vi "Digital Input Read.vi"(8 "error in (no error)":errorcluster, 11 "NI Digital Input in":refnum<class "NI Digital Input.lvclass">) -> (0 "error out":errorcluster, 2 "data":bool[](array[boolean]), 3 "NI Digital Input out":refnum<class "NI Digital Input.lvclass">)   [LabVIEW 2023, in "HardwareAbstractionLayer_LVOOP.lvlib" / "NI Digital Input.lvclass"]
uses:
  NI Digital Input.lvclass
  NI Digital Input.lvclass/NI Digital Input.ctl
  <vilib>/DAQmx/read.llb/DAQmx Read (Digital 1D Bool NChan 1Samp 1Line).vi
  <vilib>/DAQmx/miscellaneous.llb/DAQmx Fill In Error Info.vi
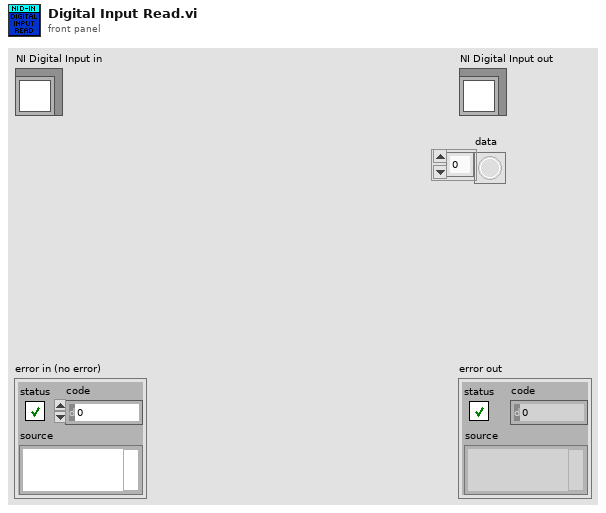
[diagram p1: front panel]
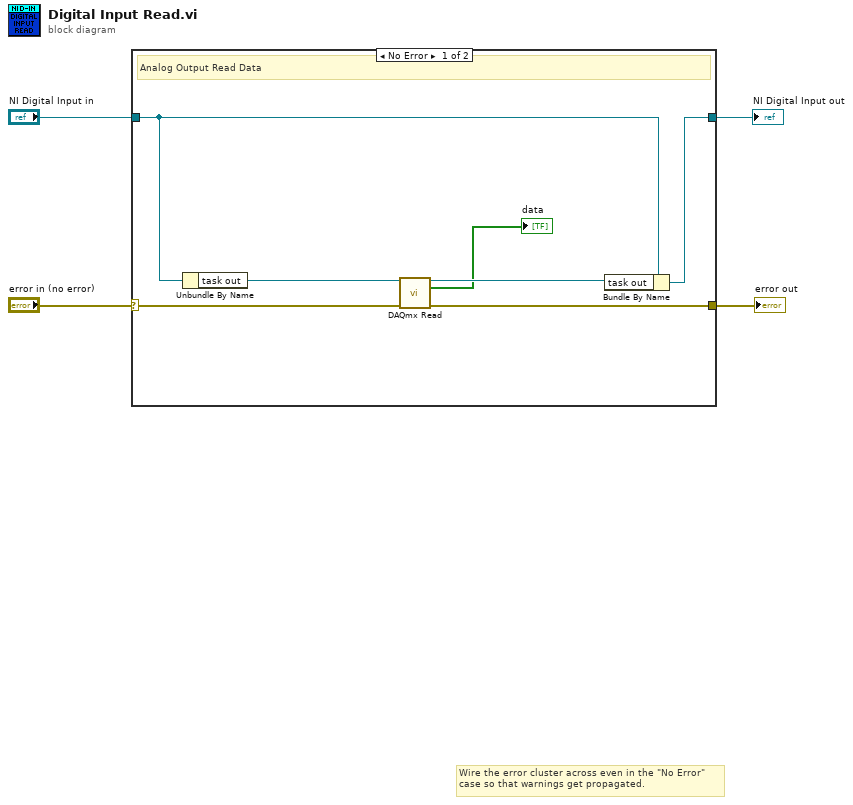
[diagram p0: block diagram]
diagram:
  # "Wire the error cluster across even in the \"No Error\"\ncase so that warnings get propagated."
  n1 = case shown="No Error" "error in (no error)" {
    selector: "error in (no error)" -> [w11 w13]
    tunnel: [w10 w13] -> w3
    tunnel: [w7 w12] -> w1
    tunnel: "NI Digital Input in" -> [w8 w12]
    frame No Error {
      # "Analog Output Read Data"
      n2 = Unbundle By Name(w8) -> ("task out"=w9:refnum<k21>)
      n3 = call-poly <vilib>:"DAQmx Read.vi"("task/channels in"=w9, "error in"=w11) -> ("task out"=w6:refnum<k21>, "data"=→"data":bool[], "error out"=w10:errorcluster)  [unwired: 11 in]
      n4 = Bundle By Name(cluster=w8, "task out"=w6) -> (w7:refnum<class "NI Digital Input.lvclass">)
    }
    frame Error {
    }
  }
  "error out" <- w3
  "NI Digital Input out" <- w1
